vi "MathCad cmd.vi"(3 "Slide Refnum":refnum<vi>, 4 "Arr Refnum":refnum<vi>, 5 "MathCAD variables":T1, 6 "MathCAD cmds":T2, 7 "Str Refnum":refnum<vi>, 8 "error in":errorcluster, 9 "Clust Refnum":refnum<vi>, 10 "Num Refnum":refnum<vi>) -> (0 "first error out":errorcluster, 1 "errors":errorcluster[](array[cluster]))   [LabVIEW 2015]
uses:
  <vilib>/Utility/config.llb/NI_LVConfig.lvlib
  <vilib>/Utility/config.llb/Read Key (Boolean).vi
  MathCAD cmd.ctl
  MathCAD results ref.ctl
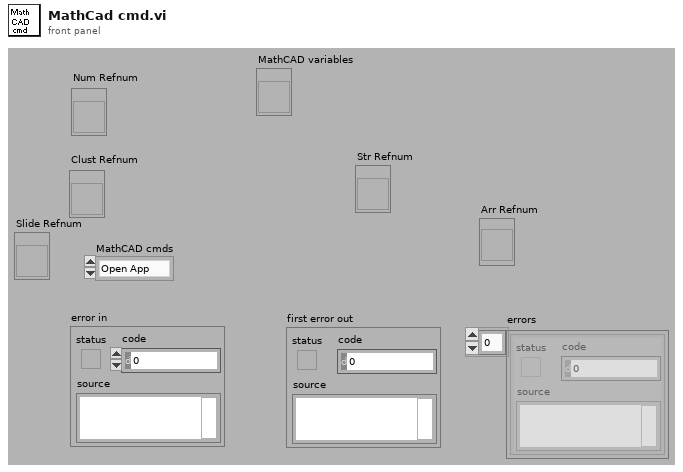
[diagram p1: front panel]
types:
  T1 = typedef "MathCAD results ref.ctl" = refnum<vi>
  T2 = typedef "MathCAD cmd.ctl" = enum16{"Open App", "Open Worksheet", "Close Worksheet", "Load Variable Ref", "Send Number", "Send Cluster", "Send Array", "Send String", "Calculate", "Get MathCAD data", "Close MathCAD"}
  T3 = typedef "NI_LVConfig.lvlib/Config Data RefNum.ctl" = refnum<k1>
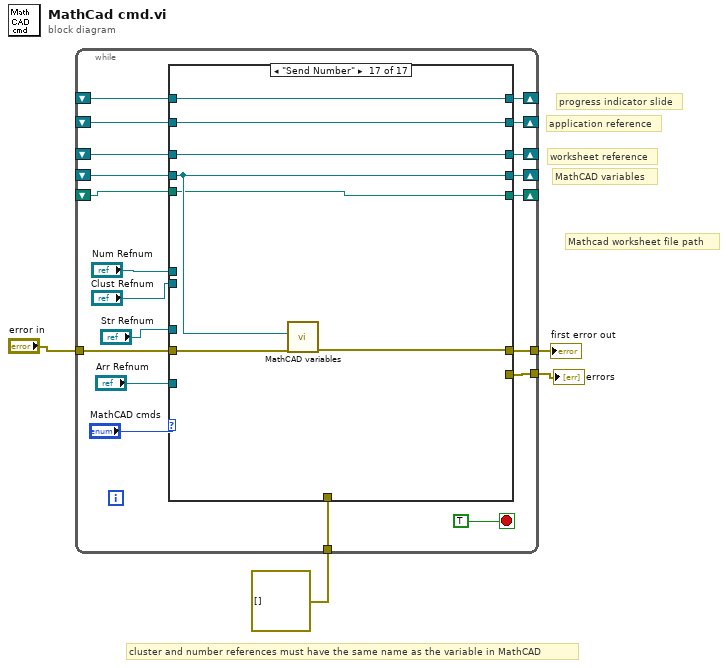
[diagram p0: block diagram]
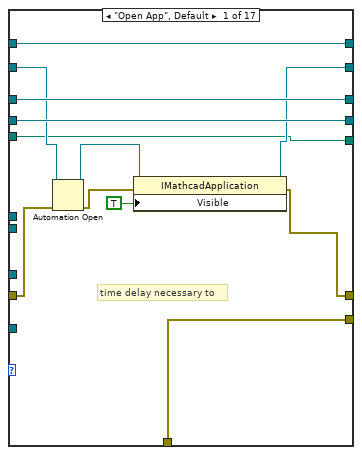
[diagram p2: hidden frame]
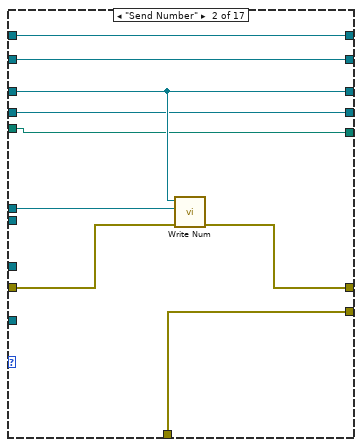
[diagram p3: hidden frame]
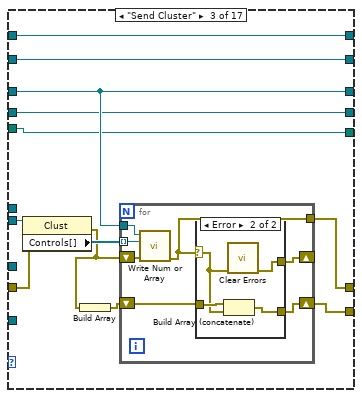
[diagram p4: hidden frame]
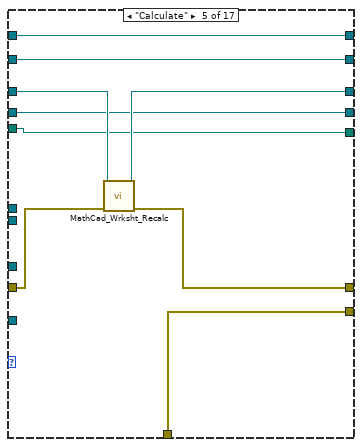
[diagram p7: hidden frame]
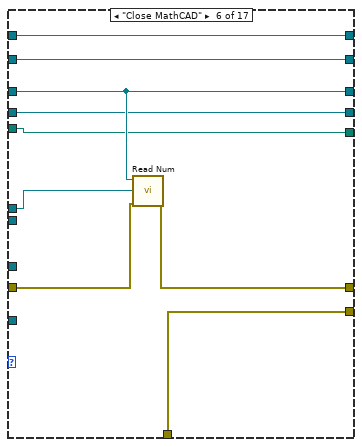
[diagram p8: hidden frame]
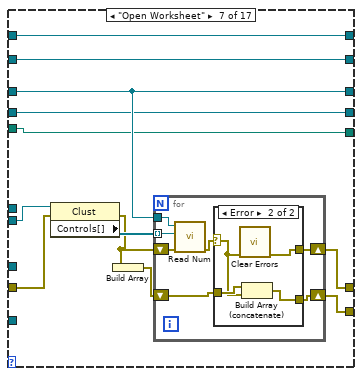
[diagram p9: hidden frame]
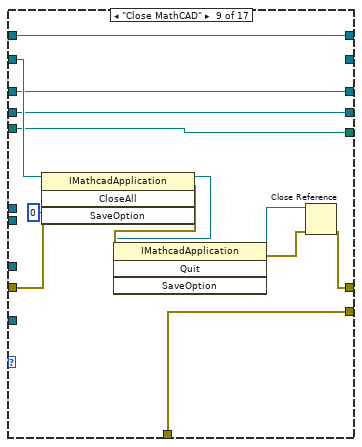
[diagram p12: hidden frame]
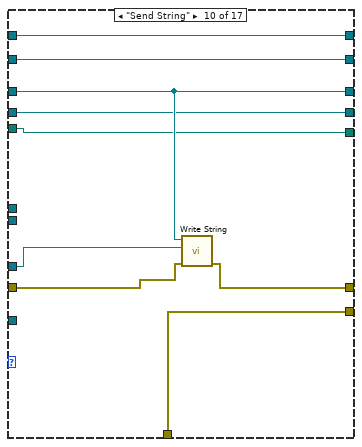
[diagram p13: hidden frame]
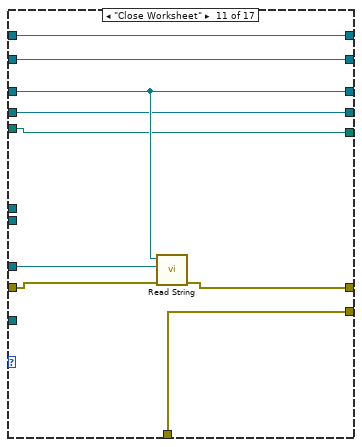
[diagram p14: hidden frame]
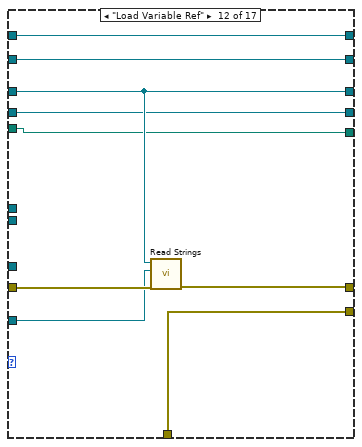
[diagram p15: hidden frame]
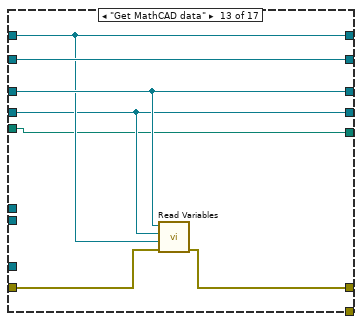
[diagram p16: hidden frame]
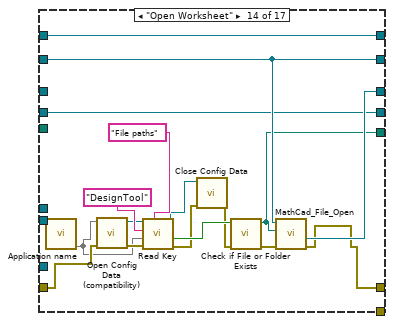
[diagram p17: hidden frame]
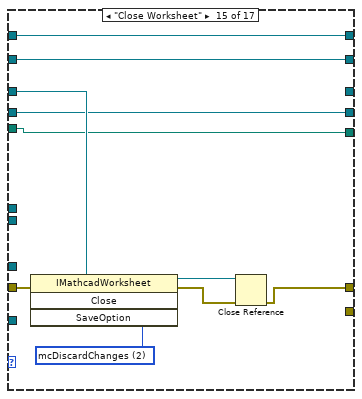
[diagram p18: hidden frame]
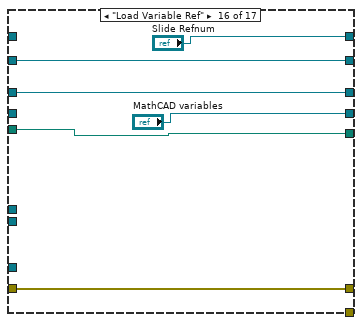
[diagram p19: hidden frame]
diagram:
  # "Mathcad worksheet file path"
  # "MathCAD variables"
  # "progress indicator slide"
  # "application reference"
  # "worksheet reference"
  # "cluster and number references must have the same name as the variable in MathCAD"
  n1 = while {
    shift-right: [w20] -> _
    shift-left: _ -> [w18]
    shift-right: [w19] -> _
    shift-left: _ -> [w17]
    tunnel: "error in" -> [w21]
    tunnel: [w22] -> w3
    tunnel: [w12] -> w2
    tunnel: errorcluster[] [] -> [w11]
    shift-right: [w10] -> _
    shift-left: _ -> [w9]
    shift-right: [w8] -> _
    shift-left: _ -> [w7]
    shift-right: [w6] -> _
    shift-left: _ -> [w5]
    stop <- TRUE stop-if-true
    n2 = case shown="\"Send Number\"" "MathCAD cmds" {
      tunnel: [w28 w42 w54 w75 w82 w94 w99 w125 w134 w147 w157 w165 w171 w176 w193 w204 w213] -> w22
      tunnel: w21 -> [w27 w44 w52 w75 w83 w95 w105 w125 w139 w148 w158 w166 w172 w184 w201 w204 w214]
      tunnel: [w29 w45 w56 w77 w86 w93 w107 w127 _ w149 w155 w167 w174 w190 w197 w205 w211] -> w20
      tunnel: [w35 w43 w55 w76 w84 w92 w104 w126 w138 w145 w154 w163 w173 w189 _ w206 w210] -> w19
      tunnel: w18 -> [w32 w45 w56 w77 w86 w93 w107 w127 w140 w149 w155 w167 w174 w190 w197 w205 w211]
      tunnel: w17 -> [w35 w43 w55 w76 w85 w92 w104 w126 w138 w145 w154 w163 w173 _ w199 w206 w210]
      tunnel: "Num Refnum" -> [_ w41 _ _ _ w91 _ _ _ _ _ _ _ _ _ _ _]
      tunnel: "Clust Refnum" -> [_ _ w53 _ _ _ w103 _ _ _ _ _ _ _ _ _ _]
      tunnel: "Str Refnum" -> [_ _ _ _ _ _ _ _ _ w146 w156 _ _ _ _ _ _]
      tunnel: "Arr Refnum" -> [_ _ _ _ _ _ _ _ _ _ _ w164 _ _ _ _ _]
      tunnel: [w36 w40 w49 w74 w81 w90 w100 w124 w137 w144 w153 w162 _ _ _ _ _] -> w12
      tunnel: w11 -> [w36 w40 _ w74 w81 w90 _ w124 w137 w144 w153 w162 _ _ _ _ _]
      tunnel: [w33 w39 w48 w73 w80 w89 w98 w123 w136 w143 w152 w161 w170 w191 w198 "Slide Refnum" w212] -> w10
      tunnel: w9 -> [w33 w39 w48 w73 w80 w89 w98 w123 w136 w143 w152 w161 w170 w191 w198 _ w212]
      tunnel: w7 -> [w34 w38 w47 w72 w79 w88 w97 w122 w135 w142 w151 w160 w169 w180 w196 _ w209]
      tunnel: [w34 w38 w47 w72 w79 w88 w97 w122 w135 w142 w151 w160 w169 w180 w196 "MathCAD variables" w209] -> w8
      tunnel: [w25 w37 w46 w71 w78 w87 w96 w121 w128 w141 w150 w159 w168 w175 w192 w202 w208] -> w6
      tunnel: w5 -> [w25 w37 w46 w71 w78 w87 w96 w121 w128 w141 w150 w159 w168 _ w192 w202 w208]
      frame "Open App", Default {
        # "time delay necessary to"
        n3 = Automation Open(error in (no error)=w27, Automation Refnum=w32) -> (Automation Refnum=w31:refnum<k7>, error out=w30:errorcluster)  [unwired: 2 in]
        n4 = property class="IMathcadApplication"(reference=w31, error in=w30, "Visible"=TRUE) -> (reference out=w29:refnum<k7>, error out=w28:errorcluster)
      }
      frame "Send Number" {
        n5 = call "Write Num.vi"("error in (no error)"=w44, "Ctl Refnum"=w41, "Worksheet Reference"=w43) -> ("error out"=w42:errorcluster)  [unwired: 8 in]
      }
      frame "Send Cluster" {
        n6 = property class="Clust"(reference=w53, error in=w52) -> (error out=w51:errorcluster, "Controls[]"=w57:refnum<vi>[])  [unwired: 1 out]
        n7 = Build Array(w51) -> (w50:errorcluster[])
        n8 = for {
          tunnel: w57 -> [w60] mode=indexing
          tunnel: w55 -> [w59]
          tunnel: [w58] -> w54
          shift-right: [w62] -> _
          shift-left: w51 -> [w61]
          shift-right: [w63] -> w49
          shift-left: w50 -> [w64]
          n9 = call "Write Num or Array.vi"("error in (no error)"=w61, "Ctl Refnum"=w60, "Worksheet Reference"=w59) -> ("error out"=w58:errorcluster)  [unwired: 8 in]
          n10 = case shown="Error" w58 {
            selector: w58 -> [w65 w68]
            tunnel: w64 -> [w66 w70]
            tunnel: [w66 w69] -> w63
            tunnel: [w65 w67] -> w62
            frame No Error {
            }
            frame Error {
              n11 = Build Array (concatenate)(w70, w68) -> (w69:errorcluster[])
              n12 = call <vilib>:"Clear Errors.vi"("error in (no error)"=w68) -> ("error out"=w67:errorcluster)  [unwired: 5 in, 1 out]
            }
          }
        }
      }
      frame "Send Array" {
      }
      frame "Calculate" {
        n13 = call "MathCad_Wrksht_Recalc.vi"("error in (no error)"=w83, "Worksheet Reference"=w85) -> ("error out"=w82:errorcluster, "Worksheet Reference"=w84:refnum<k7>)  [unwired: 8 in]
      }
      frame "Close MathCAD" {
        n14 = call "Read Num.vi"("error in (no error)"=w95, "Ctl Refnum"=w91, "Worksheet Reference"=w92) -> ("error out"=w94:errorcluster)  [unwired: 8 in]
      }
      frame "Open Worksheet" {
        n15 = property class="Clust"(reference=w103, error in=w105) -> (error out=w102:errorcluster, "Controls[]"=w106:refnum<vi>[])  [unwired: 1 out]
        n16 = Build Array(w102) -> (w101:errorcluster[])
        n17 = for {
          tunnel: w106 -> [w114] mode=indexing
          tunnel: w104 -> [w113]
          shift-right: [w109] -> w100
          shift-left: w101 -> [w110]
          shift-right: [w108] -> w99
          shift-left: w102 -> [w112]
          n18 = call "Read Num.vi"("error in (no error)"=w112, "Ctl Refnum"=w114, "Worksheet Reference"=w113) -> ("error out"=w111:errorcluster)  [unwired: 8 in]
          n19 = case shown="Error" w111 {
            selector: w111 -> [w115 w118]
            tunnel: w110 -> [w116 w120]
            tunnel: [w116 w119] -> w109
            tunnel: [w115 w117] -> w108
            frame No Error {
            }
            frame Error {
              n20 = call <vilib>:"Clear Errors.vi"("error in (no error)"=w118) -> ("error out"=w117:errorcluster)  [unwired: 5 in, 1 out]
              n21 = Build Array (concatenate)(w120, w118) -> (w119:errorcluster[])
            }
          }
        }
      }
      frame "Open App" {
      }
      frame "Close MathCAD" {
        n22 = invoke class="IMathcadApplication" method="CloseAll"(reference=w140, error in=w139, "SaveOption"=0) -> (reference out=w132:refnum<k7>, error out=w133:errorcluster)  [unwired: 1 in, 2 out]
        n23 = invoke class="IMathcadApplication" method="Quit"(reference=w132, error in=w133) -> (reference out=w131:refnum<k7>, error out=w130:errorcluster)  [unwired: 2 in, 2 out]
        n24 = Close Reference(reference=w131, error in (no error)=w130) -> (error out=w134:errorcluster)
      }
      frame "Send String" {
        n25 = call "Write String.vi"("error in (no error)"=w148, "Ctl Refnum"=w146, "Worksheet Reference"=w145) -> ("error out"=w147:errorcluster)  [unwired: 8 in]
      }
      frame "Close Worksheet" {
        n26 = call "Read String.vi"("error in (no error)"=w158, "Ctl Refnum"=w156, "Worksheet Reference"=w154) -> ("error out"=w157:errorcluster)  [unwired: 8 in]
      }
      frame "Load Variable Ref" {
        n27 = call "Read Strings.vi"("error in (no error)"=w166, "Ctl Refnum"=w164, "Worksheet Reference"=w163) -> ("error out"=w165:errorcluster)  [unwired: 8 in]
      }
      frame "Get MathCAD data" {
        n28 = call "Read Variables.vi"("error in (no error)"=w172, "Slide Refnum"=w170, "Ctl Refnum"=w169, "Worksheet Reference"=w173) -> ("error out"=w171:errorcluster)  [unwired: 7 in]
      }
      frame "Open Worksheet" {
        n29 = call "Application name.vi"() -> (0:w182)  [unwired: 4 in, 3 out]
        n30 = call <vilib>:"Open Config Data (compatibility).vi"("error in (no error)"=w184, "configuration file path"=w182) -> ("error out"=w186:errorcluster, "refnum"=w181:T3)  [unwired: 7 in, 1 out]
        n31 = call-poly <vilib>:"Read Key.vi"("section"="File paths", "error in (no error)"=w186, "default value"=w182, "key"="DesignTool", "refnum"=w181) -> ("error out"=w178:errorcluster, "value"=w187:bool, "refnum out"=w179:T3)  [unwired: 3 in, 1 out]
        n32 = call <vilib>:"Close Config Data.vi"("error in (no error)"=w178, "refnum"=w179) -> ("error out"=w177:errorcluster)  [unwired: 8 in, 1 out]
        n33 = call <vilib>:"Check if File or Folder Exists.vi"("error in (no error)"=w177, "path"=w187) -> ("error out"=w183:errorcluster, "dup path"=w175:path)  [unwired: 7 in, 1 out]
        n34 = call "MathCad_File_Open.vi"("error in (no error)"=w183, "Worksheet File"=w175, "Mathcad.IMathcadApplication"=w190) -> ("error out (no error)"=w176:errorcluster, "Worksheet Reference"=w189:refnum<k7>)  [unwired: 5 in, 2 out]
      }
      frame "Close Worksheet" {
        w200 = 2 items=["mcSaveChanges", "mcPromptToSaveChanges", "mcDiscardChanges"] ("SaveOption")
        n35 = invoke class="IMathcadWorksheet" method="Close"(reference=w199, error in=w201, "SaveOption"=w200) -> (reference out=w195:refnum<k7>, error out=w194:errorcluster)  [unwired: 1 in, 2 out]
        n36 = Close Reference(reference=w195, error in (no error)=w194) -> (error out=w193:errorcluster)
      }
      frame "Load Variable Ref" {
      }
      frame "Send Number" {
        n37 = call "MathCAD variables.vi"("error in (no error)"=w214, "MathCAD variables"=w209) -> ("error out"=w213:errorcluster)  [unwired: 8 in, 1 out]
      }
    }
  }
  "first error out" <- w3
  "errors" <- w2
